vi "Poll_tracker.vi"(0 "VISA resource name":refnum<visa-resource-name>="ASRL3::INSTR", 5 "error in (no error)":errorcluster) -> (12 "read buffer":string, 13 "Port data status":i32, 14 "VISA resource name out":refnum<visa-resource-name>, 15 "Binary mode status":string, 16 "Coordinate mode status":string, 17 "Matrix mode status":string, 18 "FPS status":i32, 19 "error out":errorcluster)   [LabVIEW 2016]
panel:
  out "Port data status index":i32
  out "Poll records":u32
  out "FPS target index":i32
  out "Matrix mode index":i32
  out "Coordinate mode index":i32
  out "Binary mode index":i32
  out "Array of tokens":string[](array[string])
  out "token index":i32
  out "Serial Settings:Number of Bytes at Serial Port":u32
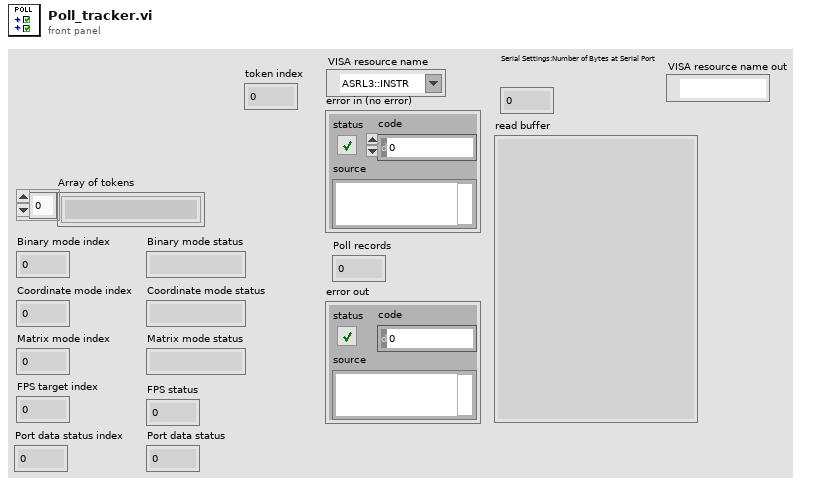
[diagram p1: front panel]
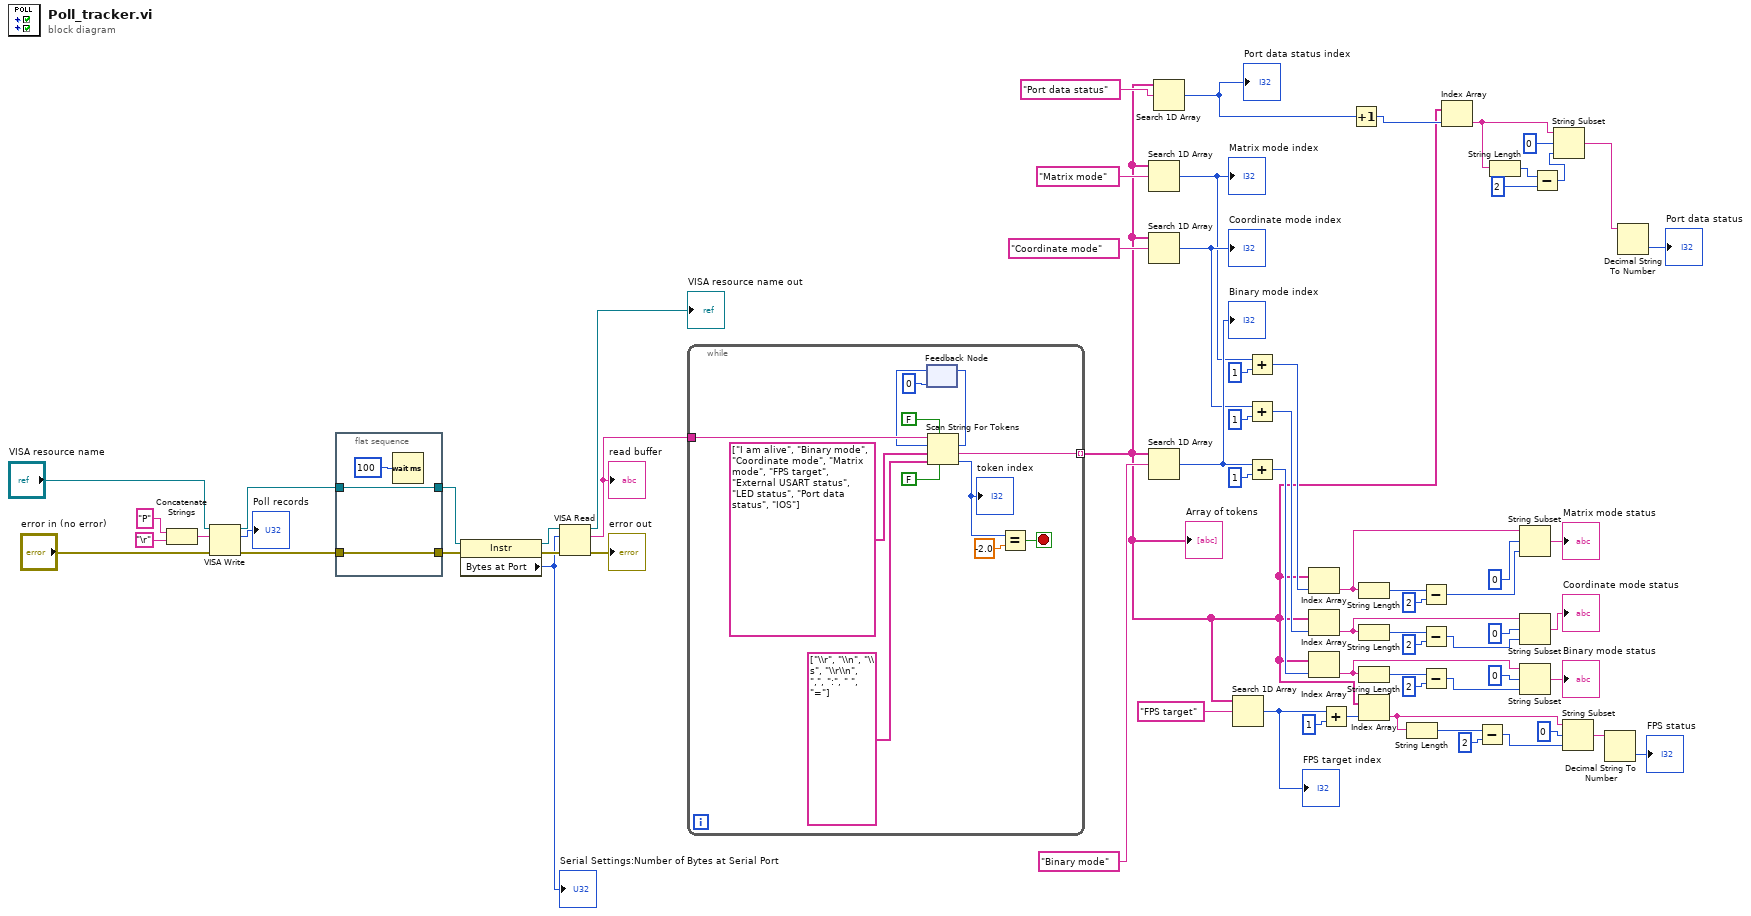
[diagram p0: block diagram]
diagram:
  n1 = Concatenate Strings("P" ("write buffer"), "\r") -> (w66:string)
  n2 = VISA Write(VISA resource name="VISA resource name", write buffer=w66, error in (no error)="error in (no error)") -> (VISA resource name out=w41:refnum<visa-resource-name>, return count=→"Poll records":u32, error out=w39:errorcluster)
  n3 = flat-sequence {
    tunnel: [w70] -> w42
    tunnel: w41 -> [w70]
    tunnel: [w69] -> w40
    tunnel: w39 -> [w69]
    frame #0 {
      n4 = Wait (ms)(milliseconds to wait=u32 100) -> ()  [unwired: 1 out]
    }
  }
  n5 = property class="Instr"(reference=w42, error in=w40) -> (reference out=w64:refnum<visa-resource-name>, error out=w63:errorcluster, "Bytes at Port"=w62:u32)
  "Serial Settings:Number of Bytes at Serial Port" <- w62
  n6 = VISA Read(VISA resource name=w64, byte count=w62, error in (no error)=w63) -> (VISA resource name out=→"VISA resource name out":refnum<visa-resource-name>, read buffer=w61:string, error out=→"error out":errorcluster)  [unwired: 1 out]
  "read buffer" <- w61
  n7 = while {
    tunnel: w61 -> [w83]
    tunnel: [w72] -> w8 mode=indexing
    stop <- w79 stop-if-true
    n8 = feedback #1(0 ("offset past token")) -> (w80:i32)
    n9 = Scan String For Tokens(4:FALSE ("use cached delim/oper data? (F)"), 5:FALSE ("allow empty tokens? (F)"), 6:string[] ["\\r", "\\n", "\\s", "\\r\\n", ",", ":", " ", "="] ("delimiters"), 7:string[] ["I am alive", "Binary mode", "Coordinate mode", "Matrix mode", "FPS target", "External USART status", "LED status", "Port data status", "IOS"] ("Tokens"), 8:w80, 9:w83) -> (0:w77:i32, 1:w72:string, 2:w81:i32)  [unwired: 1 out]
    "token index" <- w77
    n10 = feedback-in #1(w81) -> ()
    n11 = Equal?(x=w77, y=-2.0) -> (x = y?=w79:bool)
  }
  "Array of tokens" <- w8
  n12 = Search 1D Array(1D array=w8, element="Matrix mode") -> (index of element=w50:i32)  [unwired: 1 in]
  "Matrix mode index" <- w50
  n13 = Search 1D Array(1D array=w8, element="Coordinate mode") -> (index of element=w54:i32)  [unwired: 1 in]
  "Coordinate mode index" <- w54
  n14 = Search 1D Array(1D array=w8, element="Binary mode") -> (index of element=w58:i32)  [unwired: 1 in]
  "Binary mode index" <- w58
  n15 = Search 1D Array(1D array=w8, element="Port data status") -> (index of element=w10:i32)  [unwired: 1 in]
  "Port data status index" <- w10
  n16 = Search 1D Array(1D array=w8, element="FPS target") -> (index of element=w46:i32)  [unwired: 1 in]
  "FPS target index" <- w46
  n17 = Add(x=w50, y=1) -> (x+y=w51:i32)
  n18 = Add(x=w54, y=1) -> (x+y=w55:i32)
  n19 = Add(x=w58, y=1) -> (x+y=w59:i32)
  n20 = Index Array(array=w8, index=w51) -> (element=w14:string)
  n21 = Index Array(array=w8, index=w55) -> (element=w12:string)
  n22 = Index Array(array=w8, index=w59) -> (element=w35:string)
  n23 = Add(x=w46, y=1) -> (x+y=w47:i32)
  n24 = Increment(x=w10) -> (x+1=w9:i32)
  n25 = String Length(string=w14) -> (length=w29:i32)
  n26 = String Length(string=w12) -> (length=w18:i32)
  n27 = String Length(string=w35) -> (length=w34:i32)
  n28 = Index Array(array=w8, index=w47) -> (element=w13:string)
  n29 = String Length(string=w13) -> (length=w24:i32)
  n30 = Subtract(x=w29, y=2) -> (x-y=w27:i32)
  n31 = Subtract(x=w18, y=2) -> (x-y=w16:i32)
  n32 = Subtract(x=w34, y=2) -> (x-y=w32:i32)
  n33 = Index Array(array=w8, index=w9) -> (element=w7:string)
  n34 = Subtract(x=w24, y=2) -> (x-y=w22:i32)
  n35 = String Length(string=w7) -> (length=w6:i32)
  n36 = String Subset(string=w14, offset (0)=0, length (rest)=w27) -> (substring=→"Matrix mode status":string)
  n37 = String Subset(string=w12, offset (0)=0, length (rest)=w16) -> (substring=→"Coordinate mode status":string)
  n38 = String Subset(string=w35, offset (0)=0, length (rest)=w32) -> (substring=→"Binary mode status":string)
  n39 = Subtract(x=w6, y=2) -> (x-y=w4:i32)
  n40 = String Subset(string=w7, offset (0)=0, length (rest)=w4) -> (substring=w2:string)
  n41 = String Subset(string=w13, offset (0)=0, length (rest)=w22) -> (substring=w21:string)
  n42 = Decimal String To Number(string=w21) -> (number=→"FPS status":i32)  [unwired: 2 in, 1 out]
  n43 = Decimal String To Number(string=w2) -> (number=→"Port data status":i32)  [unwired: 2 in, 1 out]
